vi "Intellirupter_sensor_calibrated.vi"() -> ()   [LabVIEW 2016]
uses:
  <vilib>/rvi/Emulation/niFpgaGetClockAttributes.vi
  <vilib>/rvi/Emulation/niFpgaSctlEmulationGetInTimedLoop.vi
  <vilib>/rvi/Emulation/niFpgaEmulationReportErrorSimple.vi
  <vilib>/rvi/eio/common/nirviEmuTemplateMethod_errors.vi
  <vilib>/rvi/Emulation/niFpgaProcessEmulError.vi
  <vilib>/rvi/Emulation/niFpgaCriticalErrorInLSC.vi
  <vilib>/eio/EIONode/EIONode.xnode
panel:
  out "phase (pi) VR":fxp<+/-,32,1> format="%.32g"
  out "frequency VR":fxp<+,32,8> format="%.27g"
  out "phase (pi) VL":fxp<+/-,32,1> format="%.32g"
  out "frequency VL":fxp<+,32,8> format="%.27g"
  in  "I scale factor":fxp<+/-,26,5>
  in  "I offset":fxp<+/-,52,10>
  in  "V offset":fxp<+/-,52,10>
  in  "V scale factor":fxp<+/-,26,5>
  out "I8 B":fxp<+/-,53,11>
  out "I8 A":fxp<+/-,53,11>
  out "V8R CA":fxp<+/-,53,11>
  out "V8R BC":fxp<+/-,53,11>
  out "V8R AB":fxp<+/-,53,11>
  out "V5R CA":fxp<+/-,53,11>
  out "V5R BC":fxp<+/-,53,11>
  out "V5R AB":fxp<+/-,53,11>
  out "I5 B":fxp<+/-,53,11>
  out "I5 A":fxp<+/-,53,11>
  out "V5L CA":fxp<+/-,53,11>
  out "V5L BC":fxp<+/-,53,11>
  out "V5L AB":fxp<+/-,53,11>
  out "V4L CA":fxp<+/-,53,11>
  out "V4L BC":fxp<+/-,53,11>
  out "V4L AB":fxp<+/-,53,11>
  out "I4 C":fxp<+/-,53,11>
  out "I4 B":fxp<+/-,53,11>
  out "I4 A":fxp<+/-,53,11>
  out "V4R CA":fxp<+/-,53,11>
  out "V4R BC":fxp<+/-,53,11>
  out "V4R AB":fxp<+/-,53,11>
  out "V2L CA":fxp<+/-,53,11>
  out "V2L BC":fxp<+/-,53,11>
  out "V2L AB":fxp<+/-,53,11>
  out "I2 C":fxp<+/-,53,11>
  out "I5 C":fxp<+/-,53,11>
  out "I2 B":fxp<+/-,53,11>
  out "I2 A":fxp<+/-,53,11>
  out "V2R CA":fxp<+/-,53,11>
  out "V2R BC":fxp<+/-,53,11>
  out "V2R AB":fxp<+/-,53,11>
  out "V7R CA":fxp<+/-,53,11>
  out "V7R BC":fxp<+/-,53,11>
  out "V7R AB":fxp<+/-,53,11>
  out "I8 C":fxp<+/-,53,11>
  out "V8L CA":fxp<+/-,53,11>
  out "V8L BC":fxp<+/-,53,11>
  out "V8L AB":fxp<+/-,53,11>
  out "I7 C":fxp<+/-,53,11>
  out "I7 B":fxp<+/-,53,11> format="%.46g"
  out "I7 A":fxp<+/-,53,11> format="%.46g"
  out "V7L CA":fxp<+/-,53,11> format="%.46g"
  out "V7L BC":fxp<+/-,53,11> format="%.46g"
  out "V7L AB":fxp<+/-,53,11> format="%.46g"
  out "V6R CA":fxp<+/-,53,11> format="%.46g"
  out "V6R BC":fxp<+/-,53,11> format="%.46g"
  out "V6R AB":fxp<+/-,53,11> format="%.46g"
  out "I6 C":fxp<+/-,53,11> format="%.46g"
  out "I6 B":fxp<+/-,53,11> format="%.46g"
  out "I6 A":fxp<+/-,53,11> format="%.46g"
  out "V6L CA":fxp<+/-,53,11> format="%.46g"
  out "V6L BC":fxp<+/-,53,11> format="%.46g"
  out "V6L AB":fxp<+/-,53,11> format="%.46g"
  out "V3L CA":fxp<+/-,53,11> format="%.46g"
  out "V3L BC":fxp<+/-,53,11>
  out "V3L AB":fxp<+/-,53,11> format="%.46g"
  out "I3 C":fxp<+/-,53,11> format="%.46g"
  out "I3 B":fxp<+/-,53,11> format="%.46g"
  out "I3 A":fxp<+/-,53,11> format="%.46g"
  out "V3R CA":fxp<+/-,53,11>
  out "V3R BC":fxp<+/-,53,11> format="%.46g"
  out "V3R AB":fxp<+/-,53,11>
  out "V1L CA":fxp<+/-,53,11>
  out "V1L BC":fxp<+/-,53,11>
  out "V1L AB":fxp<+/-,53,11>
  out "I1 C":fxp<+/-,53,11> format="%.46g"
  out "I1 B":fxp<+/-,53,11>
  out "I1 A":fxp<+/-,53,11> format="%.46g"
  out "V1R CA":fxp<+/-,53,11>
  out "V1R BC":fxp<+/-,53,11>
  out "V1R AB":fxp<+/-,53,11>
  in  "Count(ticks)":u32=100
  in  "Relay7":bool
  in  "Relay8":bool
  in  "Relay6":bool
  in  "Relay5":bool
  in  "Relay3":bool
  in  "Relay4":bool
  in  "Relay1":bool
  in  "Relay2":bool
types:
  T1 = cluster{"V2R AB":fxp<+/-,53,11>, "V2R BC":fxp<+/-,53,11>}
  T2 = cluster{"V2L AB":fxp<+/-,53,11>, "V2L BC":fxp<+/-,53,11>}
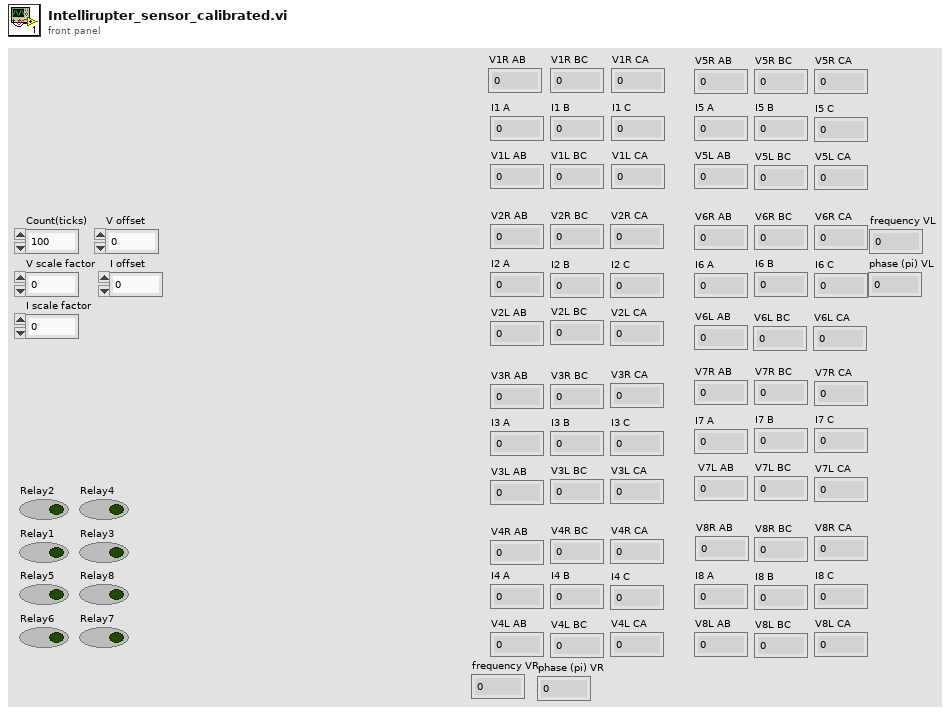
[diagram p1: front panel]
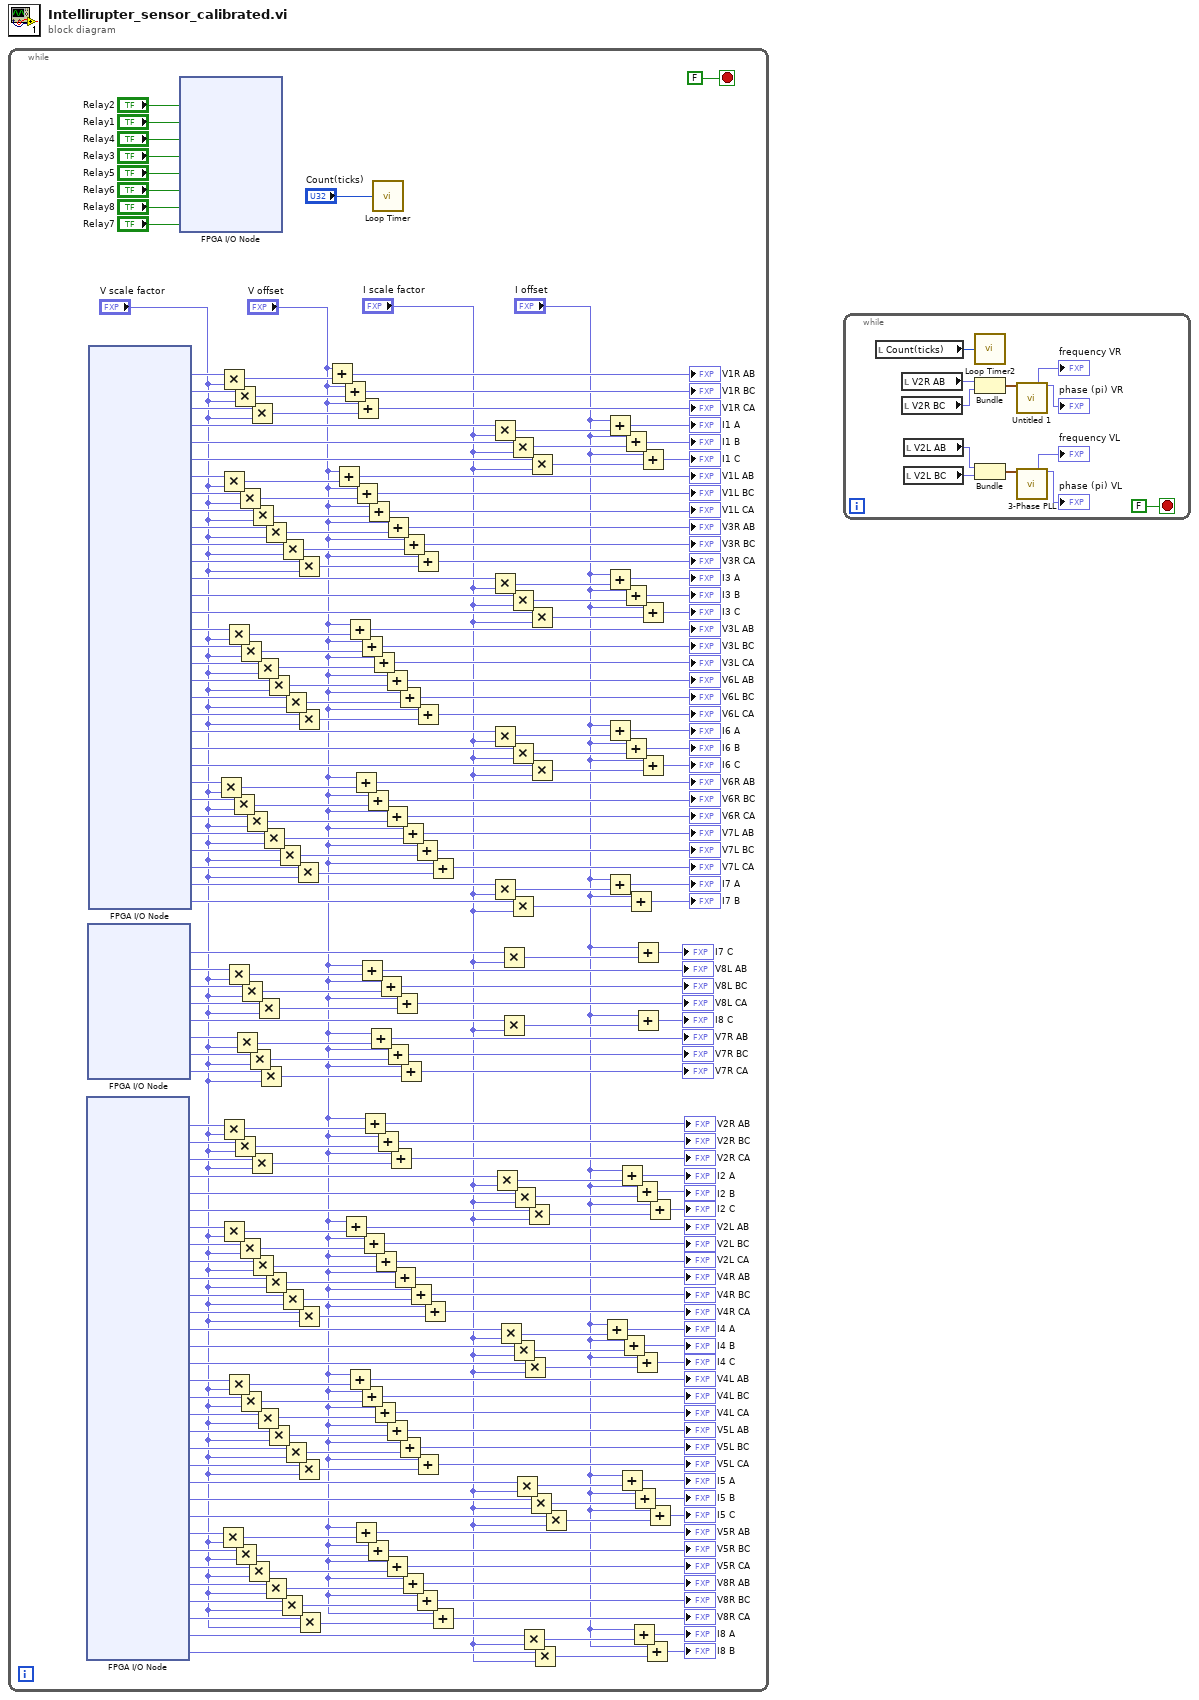
[diagram p0: block diagram]
diagram:
  n1 = while {
    stop <- FALSE stop-if-true
    n2 = xnode "FPGA I/O Node"() -> ("Mod7/AI0"=w69:fxp<+/-,26,5>, "Mod7/AI1"=w68:fxp<+/-,26,5>, "Mod7/AI2"=w67:fxp<+/-,26,5>, "Mod7/AI3"=w66:fxp<+/-,26,5>, "Mod7/AI4"=w65:fxp<+/-,26,5>, "Mod7/AI5"=w64:fxp<+/-,26,5>, "Mod7/AI6"=w63:fxp<+/-,26,5>, "Mod7/AI7"=w62:fxp<+/-,26,5>, "Mod7/AI8"=w61:fxp<+/-,26,5>, "Mod7/AI9"=w60:fxp<+/-,26,5>, "Mod7/AI10"=w59:fxp<+/-,26,5>, "Mod7/AI11"=w58:fxp<+/-,26,5>, "Mod7/AI12"=w57:fxp<+/-,26,5>, "Mod7/AI13"=w56:fxp<+/-,26,5>, "Mod7/AI14"=w55:fxp<+/-,26,5>, "Mod7/AI15"=w54:fxp<+/-,26,5>, "Mod7/AI16"=w53:fxp<+/-,26,5>, "Mod7/AI17"=w52:fxp<+/-,26,5>, "Mod7/AI18"=w51:fxp<+/-,26,5>, "Mod7/AI19"=w50:fxp<+/-,26,5>, "Mod7/AI20"=w49:fxp<+/-,26,5>, "Mod7/AI21"=w48:fxp<+/-,26,5>, "Mod7/AI22"=w47:fxp<+/-,26,5>, "Mod7/AI23"=w46:fxp<+/-,26,5>, "Mod7/AI24"=w45:fxp<+/-,26,5>, "Mod7/AI25"=w44:fxp<+/-,26,5>, "Mod7/AI26"=w43:fxp<+/-,26,5>, "Mod7/AI27"=w42:fxp<+/-,26,5>, "Mod7/AI28"=w41:fxp<+/-,26,5>, "Mod7/AI29"=w40:fxp<+/-,26,5>, "Mod7/AI30"=w39:fxp<+/-,26,5>, "Mod7/AI31"=w38:fxp<+/-,26,5>)  [unwired: 32 in, 32 out]
    n3 = xnode "FPGA I/O Node"() -> ("Mod5/AI20"=w116:fxp<+/-,26,5>, "Mod5/AI1"=w115:fxp<+/-,26,5>, "Mod5/AI2"=w114:fxp<+/-,26,5>, "Mod5/AI3"=w113:fxp<+/-,26,5>, "Mod5/AI0"=w112:fxp<+/-,26,5>, "Mod5/AI21"=w111:fxp<+/-,26,5>, "Mod5/AI22"=w110:fxp<+/-,26,5>, "Mod5/AI23"=w109:fxp<+/-,26,5>)  [unwired: 8 in, 8 out]
    n4 = xnode "FPGA I/O Node"() -> ("Mod1/AI0"=w220:fxp<+/-,26,5>, "Mod1/AI1"=w219:fxp<+/-,26,5>, "Mod1/AI2"=w218:fxp<+/-,26,5>, "Mod1/AI3"=w217:fxp<+/-,26,5>, "Mod1/AI4"=w205:fxp<+/-,26,5>, "Mod1/AI5"=w206:fxp<+/-,26,5>, "Mod1/AI6"=w207:fxp<+/-,26,5>, "Mod1/AI7"=w208:fxp<+/-,26,5>, "Mod1/AI8"=w209:fxp<+/-,26,5>, "Mod1/AI9"=w210:fxp<+/-,26,5>, "Mod1/AI10"=w211:fxp<+/-,26,5>, "Mod1/AI11"=w212:fxp<+/-,26,5>, "Mod1/AI12"=w213:fxp<+/-,26,5>, "Mod1/AI13"=w214:fxp<+/-,26,5>, "Mod1/AI14"=w215:fxp<+/-,26,5>, "Mod1/AI15"=w216:fxp<+/-,26,5>, "Mod1/AI16"=w172:fxp<+/-,26,5>, "Mod1/AI17"=w140:fxp<+/-,26,5>, "Mod1/AI18"=w139:fxp<+/-,26,5>, "Mod1/AI19"=w138:fxp<+/-,26,5>, "Mod1/AI20"=w137:fxp<+/-,26,5>, "Mod1/AI21"=w136:fxp<+/-,26,5>, "Mod1/AI22"=w135:fxp<+/-,26,5>, "Mod1/AI23"=w134:fxp<+/-,26,5>, "Mod1/AI24"=w133:fxp<+/-,26,5>, "Mod1/AI25"=w132:fxp<+/-,26,5>, "Mod1/AI26"=w131:fxp<+/-,26,5>, "Mod1/AI27"=w130:fxp<+/-,26,5>, "Mod1/AI28"=w129:fxp<+/-,26,5>, "Mod1/AI29"=w128:fxp<+/-,26,5>, "Mod1/AI30"=w127:fxp<+/-,26,5>, "Mod1/AI31"=w126:fxp<+/-,26,5>)  [unwired: 32 in, 32 out]
    n5 = xnode "FPGA I/O Node"("Mod6/DO0"="Relay2", "Mod6/DO1"="Relay1", "Mod6/DO2"="Relay4", "Mod6/DO3"="Relay3", "Mod6/DO4"="Relay5", "Mod6/DO5"="Relay6", "Mod6/DO6"="Relay8", "Mod6/DO7"="Relay7") -> ()  [unwired: 8 in, 8 out]
    n6 = Multiply(x=w133, y="V scale factor") -> (x*y=w166:fxp<+/-,52,10>)
    n7 = Multiply(x=w45, y="V scale factor") -> (x*y=w91:fxp<+/-,52,10>)
    n8 = Multiply(x=w220, y="V scale factor") -> (x*y=w204:fxp<+/-,52,10>)
    n9 = Multiply(x=w207, y="V scale factor") -> (x*y=w187:fxp<+/-,52,10>)
    n10 = Multiply(x=w69, y="V scale factor") -> (x*y=w70:fxp<+/-,52,10>)
    n11 = Multiply(x=w63, y="V scale factor") -> (x*y=w80:fxp<+/-,52,10>)
    n12 = Multiply(x=w216, y="V scale factor") -> (x*y=w196:fxp<+/-,52,10>)
    n13 = Multiply(x=w115, y="V scale factor") -> (x*y=w125:fxp<+/-,52,10>)
    n14 = Multiply(x=w54, y="V scale factor") -> (x*y=w77:fxp<+/-,52,10>)
    n15 = Multiply(x=w132, y="V scale factor") -> (x*y=w160:fxp<+/-,52,10>)
    n16 = Multiply(x=w219, y="V scale factor") -> (x*y=w202:fxp<+/-,52,10>)
    n17 = Multiply(x=w68, y="V scale factor") -> (x*y=w71:fxp<+/-,52,10>)
    n18 = Multiply(x=w44, y="V scale factor") -> (x*y=w97:fxp<+/-,52,10>)
    n19 = Multiply(x=w111, y="V scale factor") -> (x*y=w120:fxp<+/-,52,10>)
    n20 = Multiply(x=w208, y="V scale factor") -> (x*y=w185:fxp<+/-,52,10>)
    n21 = Multiply(x=w62, y="V scale factor") -> (x*y=w81:fxp<+/-,52,10>)
    n22 = Multiply(x=w172, y="V scale factor") -> (x*y=w173:fxp<+/-,52,10>)
    n23 = Multiply(x=w53, y="V scale factor") -> (x*y=w86:fxp<+/-,52,10>)
    n24 = Multiply(x=w114, y="V scale factor") -> (x*y=w124:fxp<+/-,52,10>)
    n25 = Multiply(x=w131, y="V scale factor") -> (x*y=w161:fxp<+/-,52,10>)
    n26 = Multiply(x=w43, y="V scale factor") -> (x*y=w96:fxp<+/-,52,10>)
    n27 = Multiply(x=w110, y="V scale factor") -> (x*y=w119:fxp<+/-,52,10>)
    n28 = Multiply(x=w218, y="V scale factor") -> (x*y=w201:fxp<+/-,52,10>)
    n29 = Multiply(x=w67, y="V scale factor") -> (x*y=w72:fxp<+/-,52,10>)
    n30 = Multiply(x=w209, y="V scale factor") -> (x*y=w199:fxp<+/-,52,10>)
    n31 = Multiply(x=w61, y="V scale factor") -> (x*y=w74:fxp<+/-,52,10>)
    n32 = Multiply(x=w140, y="V scale factor") -> (x*y=w157:fxp<+/-,52,10>)
    n33 = Multiply(x=w52, y="V scale factor") -> (x*y=w100:fxp<+/-,52,10>)
    n34 = Multiply(x=w113, y="V scale factor") -> (x*y=w121:fxp<+/-,52,10>)
    n35 = Multiply(x=w109, y="V scale factor") -> (x*y=w118:fxp<+/-,52,10>)
    n36 = Multiply(x=w130, y="V scale factor") -> (x*y=w167:fxp<+/-,52,10>)
    n37 = Multiply(x=w210, y="V scale factor") -> (x*y=w198:fxp<+/-,52,10>)
    n38 = Multiply(x=w60, y="V scale factor") -> (x*y=w75:fxp<+/-,52,10>)
    n39 = Multiply(x=w42, y="V scale factor") -> (x*y=w90:fxp<+/-,52,10>)
    n40 = Multiply(x=w139, y="V scale factor") -> (x*y=w158:fxp<+/-,52,10>)
    n41 = Multiply(x=w51, y="V scale factor") -> (x*y=w99:fxp<+/-,52,10>)
    n42 = Multiply(x=w129, y="V scale factor") -> (x*y=w162:fxp<+/-,52,10>)
    n43 = Multiply(x=w41, y="V scale factor") -> (x*y=w95:fxp<+/-,52,10>)
    n44 = Multiply(x=w211, y="V scale factor") -> (x*y=w182:fxp<+/-,52,10>)
    n45 = Multiply(x=w59, y="V scale factor") -> (x*y=w82:fxp<+/-,52,10>)
    n46 = Multiply(x=w138, y="V scale factor") -> (x*y=w154:fxp<+/-,52,10>)
    n47 = Multiply(x=w50, y="V scale factor") -> (x*y=w101:fxp<+/-,52,10>)
    n48 = Multiply(x=w128, y="V scale factor") -> (x*y=w168:fxp<+/-,52,10>)
    n49 = Multiply(x=w212, y="V scale factor") -> (x*y=w197:fxp<+/-,52,10>)
    n50 = Multiply(x=w137, y="V scale factor") -> (x*y=w163:fxp<+/-,52,10>)
    n51 = Multiply(x=w58, y="V scale factor") -> (x*y=w76:fxp<+/-,52,10>)
    n52 = Multiply(x=w49, y="V scale factor") -> (x*y=w94:fxp<+/-,52,10>)
    n53 = Multiply(x=w40, y="V scale factor") -> (x*y=w89:fxp<+/-,52,10>)
    n54 = Add(x="V offset", y=w204) -> (x+y=→"V1R AB":fxp<+/-,53,11>)
    n55 = Add(x="V offset", y=w187) -> (x+y=→"V1L AB":fxp<+/-,53,11>)
    n56 = Add(x="V offset", y=w202) -> (x+y=→"V1R BC":fxp<+/-,53,11>)
    n57 = Add(x="V offset", y=w80) -> (x+y=→"V2L AB":fxp<+/-,53,11>)
    n58 = Add(x="V offset", y=w196) -> (x+y=→"V3L AB":fxp<+/-,53,11>)
    n59 = Add(x="V offset", y=w77) -> (x+y=→"V4L AB":fxp<+/-,53,11>)
    n60 = Add(x="V offset", y=w166) -> (x+y=→"V6R AB":fxp<+/-,53,11>)
    n61 = Add(x="V offset", y=w91) -> (x+y=→"V5R AB":fxp<+/-,53,11>)
    n62 = Add(x="V offset", y=w185) -> (x+y=→"V1L BC":fxp<+/-,53,11>)
    n63 = Add(x="V offset", y=w201) -> (x+y=→"V1R CA":fxp<+/-,53,11>)
    n64 = Add(x="V offset", y=w173) -> (x+y=→"V3L BC":fxp<+/-,53,11>)
    n65 = Add(x="V offset", y=w125) -> (x+y=→"V8L AB":fxp<+/-,53,11>)
    n66 = Add(x="V offset", y=w86) -> (x+y=→"V4L BC":fxp<+/-,53,11>)
    n67 = Add(x="V offset", y=w81) -> (x+y=→"V2L BC":fxp<+/-,53,11>)
    n68 = Add(x="V offset", y=w70) -> (x+y=→"V2R AB":fxp<+/-,53,11>)
    n69 = Add(x="V offset", y=w160) -> (x+y=→"V6R BC":fxp<+/-,53,11>)
    n70 = Add(x="V offset", y=w97) -> (x+y=→"V5R BC":fxp<+/-,53,11>)
    n71 = Add(x="V offset", y=w199) -> (x+y=→"V1L CA":fxp<+/-,53,11>)
    n72 = Add(x="V offset", y=w120) -> (x+y=→"V7R AB":fxp<+/-,53,11>)
    n73 = Add(x="V offset", y=w157) -> (x+y=→"V3L CA":fxp<+/-,53,11>)
    n74 = Add(x="V offset", y=w100) -> (x+y=→"V4L CA":fxp<+/-,53,11>)
    n75 = Add(x="V offset", y=w74) -> (x+y=→"V2L CA":fxp<+/-,53,11>)
    n76 = call "Loop Timer"("Count(Ticks)"="Count(ticks)") -> ()  [unwired: 1 out]
    n77 = Add(x="V offset", y=w71) -> (x+y=→"V2R BC":fxp<+/-,53,11>)
    n78 = Add(x="V offset", y=w124) -> (x+y=→"V8L BC":fxp<+/-,53,11>)
    n79 = Add(x="V offset", y=w158) -> (x+y=→"V6L AB":fxp<+/-,53,11>)
    n80 = Add(x="V offset", y=w161) -> (x+y=→"V6R CA":fxp<+/-,53,11>)
    n81 = Add(x="V offset", y=w99) -> (x+y=→"V5L AB":fxp<+/-,53,11>)
    n82 = Add(x="V offset", y=w96) -> (x+y=→"V5R CA":fxp<+/-,53,11>)
    n83 = Add(x="V offset", y=w198) -> (x+y=→"V3R AB":fxp<+/-,53,11>)
    n84 = Add(x="V offset", y=w119) -> (x+y=→"V7R BC":fxp<+/-,53,11>)
    n85 = Add(x="V offset", y=w72) -> (x+y=→"V2R CA":fxp<+/-,53,11>)
    n86 = Add(x="V offset", y=w75) -> (x+y=→"V4R AB":fxp<+/-,53,11>)
    n87 = Add(x="V offset", y=w121) -> (x+y=→"V8L CA":fxp<+/-,53,11>)
    n88 = Add(x="V offset", y=w154) -> (x+y=→"V6L BC":fxp<+/-,53,11>)
    n89 = Add(x="V offset", y=w101) -> (x+y=→"V5L BC":fxp<+/-,53,11>)
    n90 = Add(x="V offset", y=w118) -> (x+y=→"V7R CA":fxp<+/-,53,11>)
    n91 = Add(x="V offset", y=w167) -> (x+y=→"V7L AB":fxp<+/-,53,11>)
    n92 = Add(x="V offset", y=w90) -> (x+y=→"V8R AB":fxp<+/-,53,11>)
    n93 = Add(x="V offset", y=w182) -> (x+y=→"V3R BC":fxp<+/-,53,11>)
    n94 = Add(x="V offset", y=w82) -> (x+y=→"V4R BC":fxp<+/-,53,11>)
    n95 = Add(x="V offset", y=w162) -> (x+y=→"V7L BC":fxp<+/-,53,11>)
    n96 = Add(x="V offset", y=w95) -> (x+y=→"V8R BC":fxp<+/-,53,11>)
    n97 = Add(x="V offset", y=w197) -> (x+y=→"V3R CA":fxp<+/-,53,11>)
    n98 = Add(x="V offset", y=w163) -> (x+y=→"V6L CA":fxp<+/-,53,11>)
    n99 = Add(x="V offset", y=w94) -> (x+y=→"V5L CA":fxp<+/-,53,11>)
    n100 = Add(x="V offset", y=w76) -> (x+y=→"V4R CA":fxp<+/-,53,11>)
    n101 = Add(x="V offset", y=w168) -> (x+y=→"V7L CA":fxp<+/-,53,11>)
    n102 = Add(x="V offset", y=w89) -> (x+y=→"V8R CA":fxp<+/-,53,11>)
    n103 = Multiply(x=w217, y="I scale factor") -> (x*y=w192:fxp<+/-,52,10>)
    n104 = Multiply(x=w213, y="I scale factor") -> (x*y=w179:fxp<+/-,52,10>)
    n105 = Multiply(x=w136, y="I scale factor") -> (x*y=w159:fxp<+/-,52,10>)
    n106 = Multiply(x=w127, y="I scale factor") -> (x*y=w169:fxp<+/-,52,10>)
    n107 = Multiply(x=w66, y="I scale factor") -> (x*y=w78:fxp<+/-,52,10>)
    n108 = Multiply(x=w57, y="I scale factor") -> (x*y=w83:fxp<+/-,52,10>)
    n109 = Multiply(x=w116, y="I scale factor") -> (x*y=w122:fxp<+/-,52,10>)
    n110 = Multiply(x=w112, y="I scale factor") -> (x*y=w123:fxp<+/-,52,10>)
    n111 = Multiply(x=w205, y="I scale factor") -> (x*y=w200:fxp<+/-,52,10>)
    n112 = Multiply(x=w214, y="I scale factor") -> (x*y=w177:fxp<+/-,52,10>)
    n113 = Multiply(x=w135, y="I scale factor") -> (x*y=w164:fxp<+/-,52,10>)
    n114 = Multiply(x=w126, y="I scale factor") -> (x*y=w170:fxp<+/-,52,10>)
    n115 = Multiply(x=w56, y="I scale factor") -> (x*y=w84:fxp<+/-,52,10>)
    n116 = Multiply(x=w65, y="I scale factor") -> (x*y=w73:fxp<+/-,52,10>)
    n117 = Multiply(x=w48, y="I scale factor") -> (x*y=w98:fxp<+/-,52,10>)
    n118 = Multiply(x=w39, y="I scale factor") -> (x*y=w88:fxp<+/-,52,10>)
    n119 = Multiply(x=w55, y="I scale factor") -> (x*y=w85:fxp<+/-,52,10>)
    n120 = Multiply(x=w64, y="I scale factor") -> (x*y=w79:fxp<+/-,52,10>)
    n121 = Multiply(x=w47, y="I scale factor") -> (x*y=w93:fxp<+/-,52,10>)
    n122 = Multiply(x=w206, y="I scale factor") -> (x*y=w189:fxp<+/-,52,10>)
    n123 = Multiply(x=w215, y="I scale factor") -> (x*y=w175:fxp<+/-,52,10>)
    n124 = Multiply(x=w134, y="I scale factor") -> (x*y=w165:fxp<+/-,52,10>)
    n125 = Multiply(x=w38, y="I scale factor") -> (x*y=w87:fxp<+/-,52,10>)
    n126 = Multiply(x=w46, y="I scale factor") -> (x*y=w92:fxp<+/-,52,10>)
    n127 = Add(x="I offset", y=w83) -> (x+y=→"I4 A":fxp<+/-,53,11>)
    n128 = Add(x="I offset", y=w192) -> (x+y=→"I1 A":fxp<+/-,53,11>)
    n129 = Add(x="I offset", y=w179) -> (x+y=→"I3 A":fxp<+/-,53,11>)
    n130 = Add(x="I offset", y=w159) -> (x+y=→"I6 A":fxp<+/-,53,11>)
    n131 = Add(x="I offset", y=w169) -> (x+y=→"I7 A":fxp<+/-,53,11>)
    n132 = Add(x="I offset", y=w78) -> (x+y=→"I2 A":fxp<+/-,53,11>)
    n133 = Add(x="I offset", y=w98) -> (x+y=→"I5 A":fxp<+/-,53,11>)
    n134 = Add(x="I offset", y=w84) -> (x+y=→"I4 B":fxp<+/-,53,11>)
    n135 = Add(x="I offset", y=w200) -> (x+y=→"I1 B":fxp<+/-,53,11>)
    n136 = Add(x="I offset", y=w177) -> (x+y=→"I3 B":fxp<+/-,53,11>)
    n137 = Add(x="I offset", y=w164) -> (x+y=→"I6 B":fxp<+/-,53,11>)
    n138 = Add(x="I offset", y=w170) -> (x+y=→"I7 B":fxp<+/-,53,11>)
    n139 = Add(x="I offset", y=w88) -> (x+y=→"I8 A":fxp<+/-,53,11>)
    n140 = Add(x="I offset", y=w93) -> (x+y=→"I5 B":fxp<+/-,53,11>)
    n141 = Add(x="I offset", y=w73) -> (x+y=→"I2 B":fxp<+/-,53,11>)
    n142 = Add(x="I offset", y=w85) -> (x+y=→"I4 C":fxp<+/-,53,11>)
    n143 = Add(x="I offset", y=w122) -> (x+y=→"I7 C":fxp<+/-,53,11>)
    n144 = Add(x="I offset", y=w123) -> (x+y=→"I8 C":fxp<+/-,53,11>)
    n145 = Add(x="I offset", y=w189) -> (x+y=→"I1 C":fxp<+/-,53,11>)
    n146 = Add(x="I offset", y=w175) -> (x+y=→"I3 C":fxp<+/-,53,11>)
    n147 = Add(x="I offset", y=w165) -> (x+y=→"I6 C":fxp<+/-,53,11>)
    n148 = Add(x="I offset", y=w87) -> (x+y=→"I8 B":fxp<+/-,53,11>)
    n149 = Add(x="I offset", y=w79) -> (x+y=→"I2 C":fxp<+/-,53,11>)
    n150 = Add(x="I offset", y=w92) -> (x+y=→"I5 C":fxp<+/-,53,11>)
  }
  n151 = while {
    stop <- FALSE stop-if-true
    n152 = local read "Count(ticks)"() -> (w241:u32)
    n153 = local read "V2R AB"() -> (w236:fxp<+/-,53,11>)
    n154 = local read "V2R BC"() -> (w235:fxp<+/-,53,11>)
    n155 = local read "V2L AB"() -> (w240:fxp<+/-,53,11>)
    n156 = local read "V2L BC"() -> (w239:fxp<+/-,53,11>)
    n157 = call "Loop Timer2"("Count(Ticks)"=w241) -> ()  [unwired: 1 out]
    n158 = Bundle("V2R AB"=w236, "V2R BC"=w235) -> (w237:T1)  [unwired: 1 in]
    n159 = Bundle("V2L AB"=w240, "V2L BC"=w239) -> (w238:T2)  [unwired: 1 in]
    n160 = call "Untitled 1.vi"("input (line value)"=w237) -> ("frequency"=→"frequency VR":fxp<+,32,8>, "phase (pi)"=→"phase (pi) VR":fxp<+/-,32,1>)  [unwired: 11 in, 2 out]
    n161 = call "3-Phase PLL"("input (line value)"=w238) -> ("frequency"=→"frequency VL":fxp<+,32,8>, "phase (pi)"=→"phase (pi) VL":fxp<+/-,32,1>)  [unwired: 11 in, 2 out]
  }
